vi "Set Value.vi"(8 "error in (no error)":errorcluster, 10 "Value":variant, 11 "LimitType in":refnum<class "Numeric Limit.lvclass">) -> (0 "error out":errorcluster, 3 "LimitType out":refnum<class "Numeric Limit.lvclass">)   [LabVIEW 2017, in "Numeric Limit.lvclass"]
uses:
  Numeric Limit.lvclass
  Numeric Limit.ctl
  Numeric Limit.lvclass/Numeric Limit.ctl
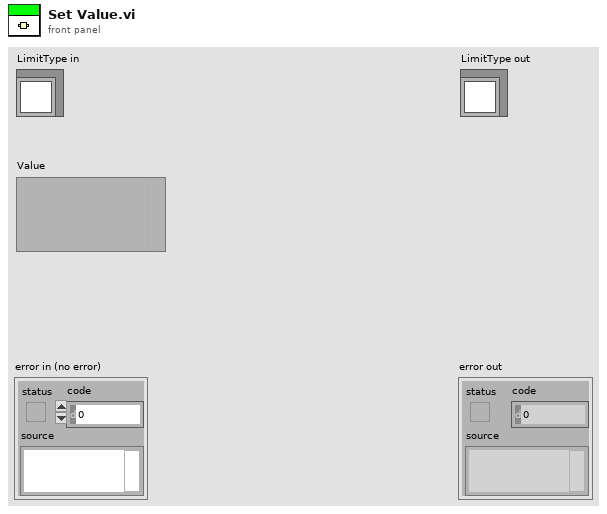
[diagram p1: front panel]
types:
  T1 = typedef "Numeric Limit.ctl" = cluster{"High Limit":dbl, "Low Limit":dbl, "Check Item":string, "Assertion HIGH":u16, "Assertion LOW":u16}
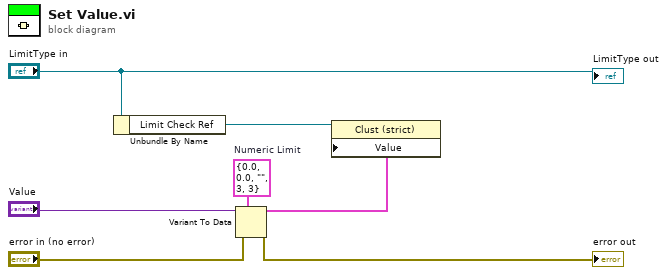
[diagram p0: block diagram]
diagram:
  w4 = T1 {"High Limit"=0.0, "Low Limit"=0.0, "Check Item"="", "Assertion HIGH"=3, "Assertion LOW"=3}  # Numeric Limit
  n1 = Unbundle By Name("LimitType in") -> ("Limit Check Ref"=w5:refnum<vi>)
  n2 = Variant To Data(error in="error in (no error)", type=w4, Variant="Value") -> (data=w3:T1, error out=→"error out":errorcluster)
  n3 = property class="Clust (strict)"(reference=w5, "Value"=w3) -> ()  [unwired: 1 in, 2 out]
  "LimitType out" <- "LimitType in"
